vi "prePurge.vi"(8 "error in":errorcluster, 9 "Boiler Simulation Controls":refnum<vi>, 10 "Boiler Controls":refnum<vi>, 11 "Boiler Status Indicators":refnum<vi>) -> (0 "error out":errorcluster, 3 "elapsedTime":dbl)   [LabVIEW 2024]
uses:
  Controls/Boiler Simulation Controls.ctl
  Controls/Boiler Status Indicators.ctl
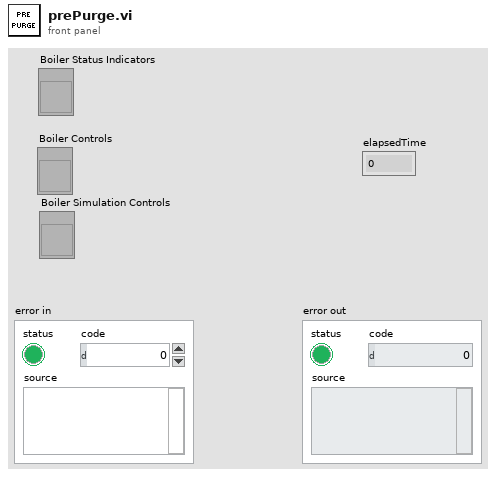
[diagram p1: front panel]
types:
  T1 = typedef "Boiler Status Indicators.ctl" = cluster{"Status":string, "Primary Fan":bool, "Natural Gas Valve":bool, "Pilot":bool, "Fuel Valve":bool, "Forced Draft Fan":bool, "Time Count":dbl}
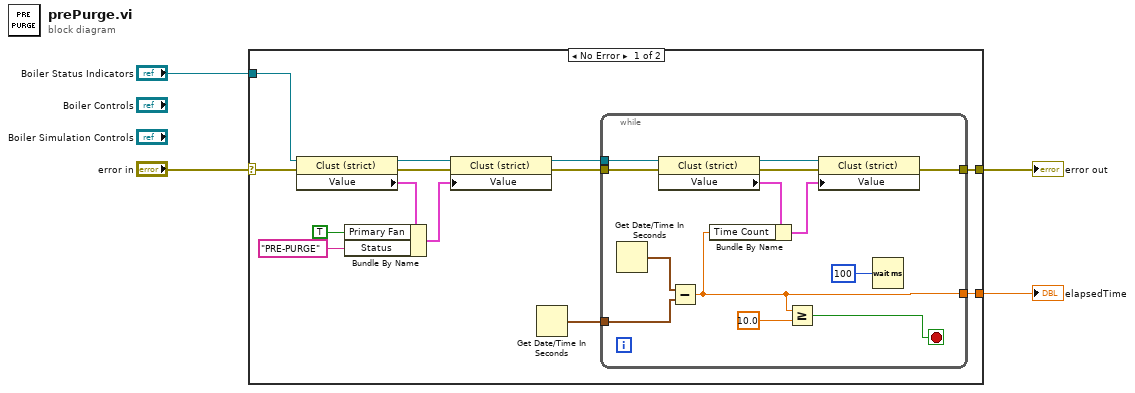
[diagram p0: block diagram]
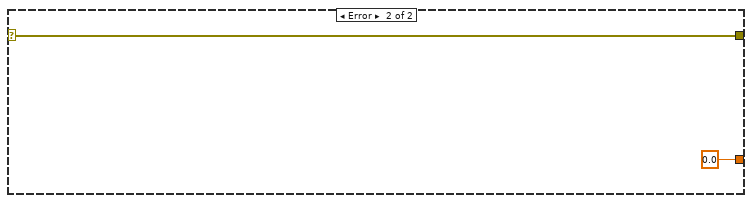
[diagram p2: hidden frame]
diagram:
  n1 = case shown="No Error" "error in" {
    selector: "error in" -> [w17 w32]
    tunnel: [w7 w32] -> w3
    tunnel: "Boiler Status Indicators" -> [w16 _]
    tunnel: [w5 0.0] -> w1
    frame No Error {
      n2 = property class="Clust (strict)"(reference=w16, error in=w17) -> (reference out=w15:refnum<vi>, error out=w14:errorcluster, "Value"=w13:T1)
      n3 = Bundle By Name(cluster=w13, "Primary Fan"=TRUE, "Status"="PRE-PURGE") -> (w12:T1)
      n4 = property class="Clust (strict)"(reference=w15, error in=w14, "Value"=w12) -> (reference out=w9:refnum<vi>, error out=w8:errorcluster)
      n5 = Get Date/Time In Seconds() -> (seconds since 1Jan1904=w6:timestamp)
      n6 = while {
        tunnel: w9 -> [w26]
        tunnel: w8 -> [w25]
        tunnel: [w24] -> w7
        tunnel: w6 -> [w22]
        tunnel: [w18] -> w5
        stop <- w20 stop-if-true
        n7 = Get Date/Time In Seconds() -> (seconds since 1Jan1904=w23:timestamp)
        n8 = property class="Clust (strict)"(reference=w26, error in=w25) -> (reference out=w27:refnum<vi>, error out=w28:errorcluster, "Value"=w29:T1)
        n9 = Subtract(x=w23, y=w22) -> (x-y=w18:dbl)
        n10 = Bundle By Name(cluster=w29, "Time Count"=w18) -> (w30:T1)
        n11 = Greater Or Equal?(x=w18, y=10.0) -> (x >= y?=w20:bool)
        n12 = property class="Clust (strict)"(reference=w27, error in=w28, "Value"=w30) -> (error out=w24:errorcluster)  [unwired: 1 out]
        n13 = Wait (ms)(milliseconds to wait=u32 100) -> ()  [unwired: 1 out]
      }
    }
    frame Error {
    }
  }
  "error out" <- w3
  "elapsedTime" <- w1
